vi "rd_getCreator.vi"(8 "error in (no error)":errorcluster, 11 "creator":string) -> (0 "error out":errorcluster, 3 "creator out":string)   [LabVIEW 2020, in "NI_ExcelFile.lvlib"]
uses:
  <vilib>/express/express shared/NI_ExcelFile/NI_ExcelFile.lvlib
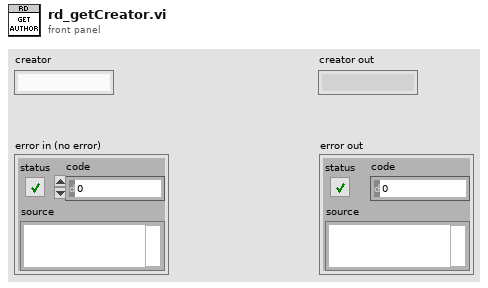
[diagram p1: front panel]
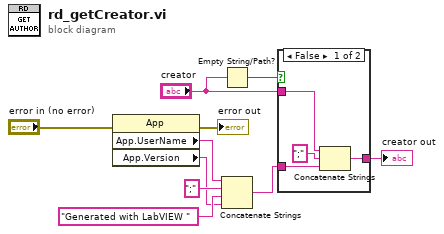
[diagram p0: block diagram]
diagram:
  n1 = property class="App"(error in="error in (no error)") -> (error out=→"error out":errorcluster, "App.UserName"=w8:string, "App.Version"=w1:string)  [unwired: 1 in, 1 out]
  n2 = Empty String/Path?(string/path="creator") -> (empty?=w5:bool)
  n3 = Concatenate Strings(w8, ";" ("string"), "Generated with LabVIEW " ("string"), w1) -> (w4:string)
  n4 = case shown="False" w5 {
    tunnel: w4 -> [w12 w15]
    tunnel: [w11 w15] -> w10
    tunnel: "creator" -> [w14 _]
    frame False {
      n5 = Concatenate Strings(w14, ";" ("string"), w12) -> (w11:string)
    }
    frame True {
    }
  }
  "creator out" <- w10
